vi "Timing.vi"(7 "Task":enum16{"Reset", "Run", "Pause"}(ring), 8 "error in (no error)":errorcluster, 11 "Time Period (s)":u32=5) -> (0 "error out":errorcluster, 1 "Timer":dbl, 2 "Period Done":bool, 3 "Elapsed Time":dbl)   [LabVIEW 2015]
doc: "FGV that keeps track of station timing. The pause task will halt a current time keeping and must be run immediately before resuming timing."
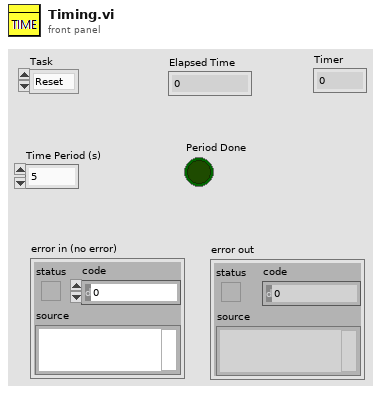
[diagram p1: front panel]
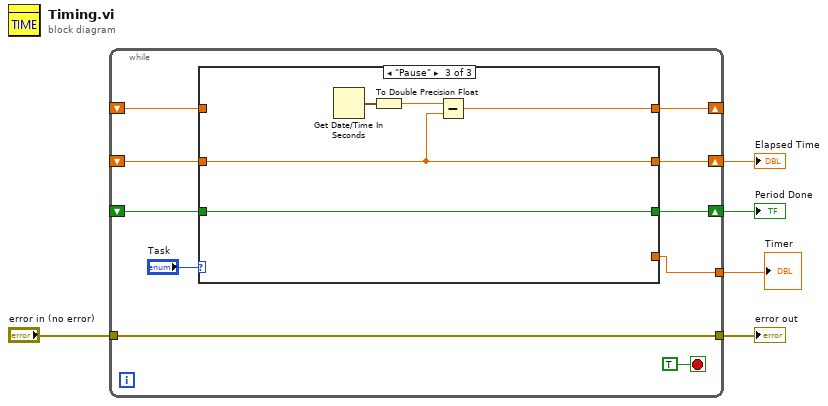
[diagram p0: block diagram]
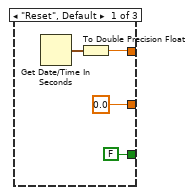
[diagram p2: hidden frame]
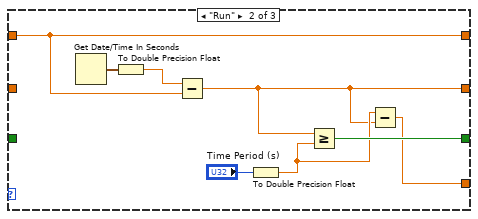
[diagram p3: hidden frame]
diagram:
  n1 = while {
    shift-right: [w13] -> _
    shift-left: _ -> [w11]
    tunnel: "error in (no error)" -> [w9]
    tunnel: [w9] -> w2
    shift-right: [w12] -> w5
    shift-left: _ -> [w7]
    shift-right: [w10] -> w4
    shift-left: _ -> [w8]
    tunnel: [w6] -> w1
    stop <- TRUE stop-if-true
    n2 = case shown="\"Pause\"" "Task" {
      tunnel: [w18 w25 w29] -> w13
      tunnel: [0.0 w21 w28] -> w12
      tunnel: w11 -> [_ w25 _]
      tunnel: [FALSE w23 w32] -> w10
      tunnel: w8 -> [_ _ w32]
      tunnel: w7 -> [_ _ w28]
      tunnel: [_ w20 _] -> w6
      frame "Reset", Default {
        n3 = Get Date/Time In Seconds() -> (seconds since 1Jan1904=w19:timestamp)
        n4 = To Double Precision Float(number=w19) -> (double precision float=w18:dbl)
      }
      frame "Run" {
        n5 = Get Date/Time In Seconds() -> (seconds since 1Jan1904=w27:timestamp)
        n6 = To Double Precision Float(number=w27) -> (double precision float=w26:dbl)
        n7 = Subtract(x=w26, y=w25) -> (x-y=w21:dbl)
        n8 = To Double Precision Float(number="Time Period (s)") -> (double precision float=w22:dbl)
        n9 = Greater Or Equal?(x=w21, y=w22) -> (x >= y?=w23:bool)
        n10 = Subtract(x=w22, y=w21) -> (x-y=w20:dbl)
      }
      frame "Pause" {
        n11 = Get Date/Time In Seconds() -> (seconds since 1Jan1904=w31:timestamp)
        n12 = To Double Precision Float(number=w31) -> (double precision float=w30:dbl)
        n13 = Subtract(x=w30, y=w28) -> (x-y=w29:dbl)
      }
    }
  }
  "Elapsed Time" <- w5
  "Period Done" <- w4
  "error out" <- w2
  "Timer" <- w1
